vi "run s4gei state mach.vi"(8 "error in (no error)":errorcluster, 11 "S4GEI in":refnum<class "S4GEI.lvclass">) -> (0 "error out":errorcluster, 3 "S4GEI out":refnum<class "S4GEI.lvclass">)   [LabVIEW 2018, in "S4GEI.lvclass"]
uses:
  S4GEI.lvclass
  S4GEI.lvclass/S4GEI.ctl
  State Machine/State Machine.lvclass
  Channel GUI/Channel.lvclass
panel:
  out "preset modes":T1
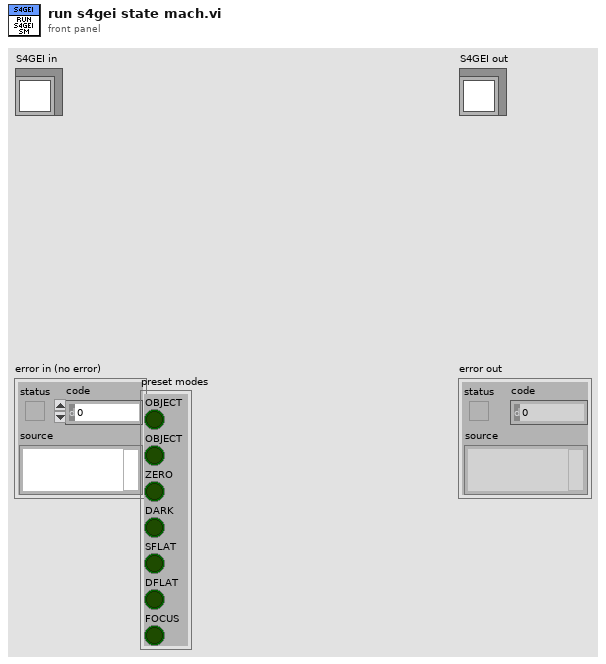
[diagram p1: front panel]
types:
  T1 = cluster{"OBJECT":bool, "OBJECT":bool, "ZERO":bool, "DARK":bool, "SFLAT":bool, "DFLAT":bool, "FOCUS":bool}
  T2 = cluster{"OBJECT":bool, "TEST":bool, "ZERO":bool, "DARK":bool, "SFLAT":bool, "DFLAT":bool, "FOCUS":bool}
  T3 = cluster{"OBJECT":string, "OBSERVER":string, "CTRLINTE":string, "PROJID":string, "SYNCMODE":string, "INSTMODE":string, "FILTER":string, "OBSTYPE":string, "GUIVRSN":string, "COMMENT":string, "broker":string, "timestamp":string, "CHANNEL 1":bool, "CHANNEL 2":bool, "CHANNEL 3":bool, "CHANNEL 4":bool, "TCSMODE":bool}
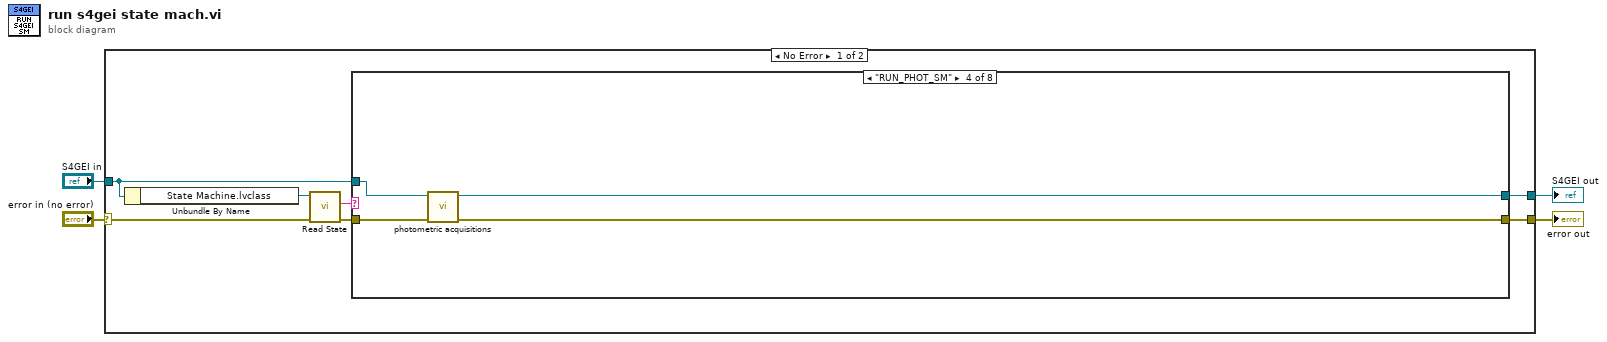
[diagram p0: block diagram]
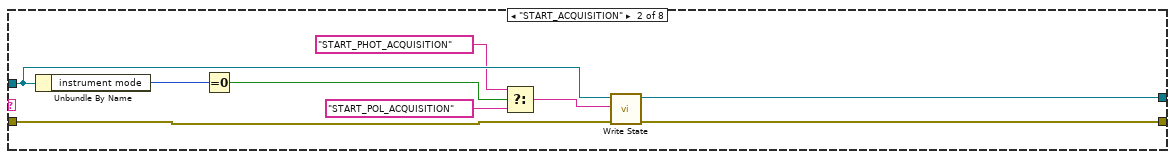
[diagram p3: hidden frame]
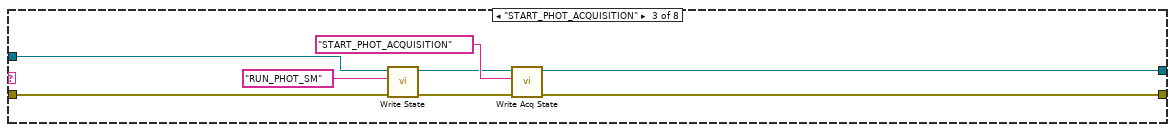
[diagram p4: hidden frame]
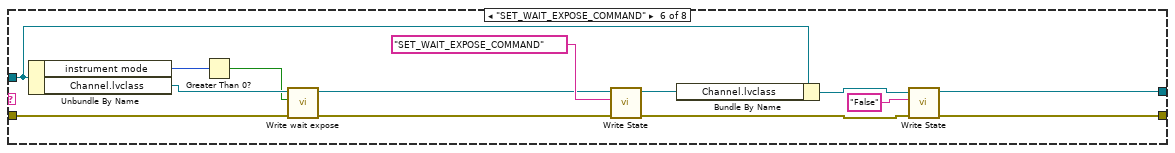
[diagram p6: hidden frame]
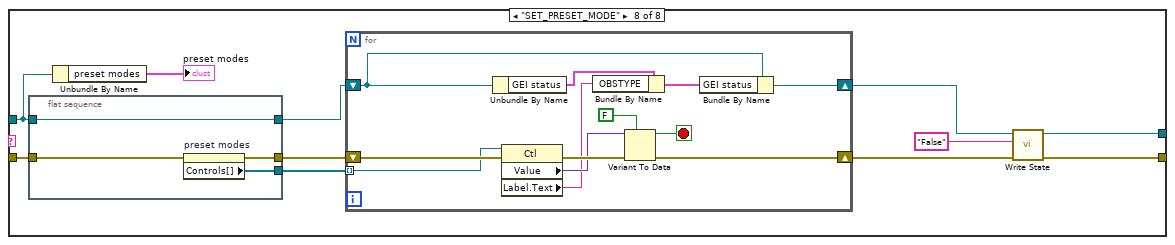
[diagram p8: hidden frame]
diagram:
  n1 = case shown="No Error" "error in (no error)" {
    selector: "error in (no error)" -> [w7 w81]
    tunnel: [w10 w81] -> w3
    tunnel: [w11 w80] -> w1
    tunnel: "S4GEI in" -> [w9 w80]
    frame No Error {
      n2 = Unbundle By Name(w9) -> ("State Machine.lvclass"=w8:refnum<class "State Machine.lvclass">)
      n3 = call-dynamic "Read State.vi"("error in (no error)"=w7, "State Machine in"=w8) -> ("error out"=w6:errorcluster, "State"=w5:string)  [unwired: 7 in, 1 out]
      n4 = case shown="\"RUN_PHOT_SM\"" w5 {
        tunnel: w9 -> [w13 w18 w27 w34 w36 w50 w52 w59]
        tunnel: w6 -> [w12 w19 w24 w31 w35 w39 w51 w58]
        tunnel: [w13 w21 w29 w33 w36 w47 w52 w56] -> w11
        tunnel: [w12 w22 w30 w32 w35 w46 w51 w57] -> w10
        frame "False", Default {
        }
        frame "START_ACQUISITION" {
          n5 = Unbundle By Name(w18) -> ("instrument mode"=w20:u16)
          n6 = Equal To 0?(x=w20) -> (x = 0?=w17:bool)
          n7 = Select(t="START_PHOT_ACQUISITION", s=w17, f="START_POL_ACQUISITION") -> (s? t:f=w15:string)
          n8 = call "Write State.vi"("error in (no error)"=w19, "State"=w15, "SPARC4_GEI in"=w18) -> ("error out"=w22:errorcluster, "SPARC4_GEI out"=w21:refnum<class "S4GEI.lvclass">)  [unwired: 7 in]
        }
        frame "START_PHOT_ACQUISITION" {
          n9 = call "Write State.vi"("error in (no error)"=w24, "State"="RUN_PHOT_SM", "SPARC4_GEI in"=w27) -> ("error out"=w25:errorcluster, "SPARC4_GEI out"=w26:refnum<class "S4GEI.lvclass">)  [unwired: 7 in]
          n10 = call "Write Acq State.vi"("error in (no error)"=w25, "State"="START_PHOT_ACQUISITION", "SPARC4_GEI in"=w26) -> ("error out"=w30:errorcluster, "SPARC4_GEI out"=w29:refnum<class "S4GEI.lvclass">)  [unwired: 7 in]
        }
        frame "RUN_PHOT_SM" {
          n11 = call "photometric acquisitions.vi"("error in (no error)"=w31, "S4GEI in"=w34) -> ("error out"=w32:errorcluster, "S4GEI out"=w33:refnum<class "S4GEI.lvclass">)  [unwired: 8 in]
        }
        frame "-------------------------" {
        }
        frame "SET_WAIT_EXPOSE_COMMAND" {
          n12 = Unbundle By Name(w50) -> ("instrument mode"=w38:u16, "Channel.lvclass"=w42:refnum<class "Channel.lvclass">)
          n13 = Greater Than 0?(x=w38) -> (x > 0?=w37:bool)
          n14 = call-dynamic "Write wait expose.vi"("error in (no error)"=w39, "wait expose"=w37, "Channel in"=w42) -> ("error out"=w40:errorcluster, "Channel out"=w41:refnum<class "Channel.lvclass">)  [unwired: 7 in]
          n15 = call "Write State.vi"("error in (no error)"=w40, "State"="SET_WAIT_EXPOSE_COMMAND", "Channel GEI in"=w41) -> ("error out"=w45:errorcluster, "Channel GEI out"=w49:refnum<class "Channel.lvclass">)  [unwired: 7 in]
          n16 = Bundle By Name(cluster=w50, "Channel.lvclass"=w49) -> (w48:refnum<class "S4GEI.lvclass">)
          n17 = call "Write State.vi"("error in (no error)"=w45, "State"="False", "SPARC4_GEI in"=w48) -> ("error out"=w46:errorcluster, "SPARC4_GEI out"=w47:refnum<class "S4GEI.lvclass">)  [unwired: 7 in]
        }
        frame "--------------------------" {
        }
        frame "SET_PRESET_MODE" {
          n18 = flat-sequence {
            tunnel: w58 -> [w65]
            tunnel: [w66] -> w63
            tunnel: w59 -> [w67]
            tunnel: [w67] -> w62
            tunnel: [w64] -> w60
            frame #0 {
              n19 = property on="preset modes" class="Clust (strict)"(error in=w65) -> (error out=w66:errorcluster, "Controls[]"=w64:refnum<vi>[])  [unwired: 1 in, 1 out]
            }
          }
          n20 = Unbundle By Name(w59) -> ("preset modes"=→"preset modes":T2)
          n21 = for {
            shift-right: [w70] -> w55
            shift-left: w62 -> [w74]
            shift-right: [w69] -> w54
            shift-left: w63 -> [w79]
            tunnel: w60 -> [w68] mode=indexing
            stop <- w75 stop-if-true
            n22 = Unbundle By Name(w74) -> ("GEI status"=w73:T3)
            n23 = property class="Ctl"(reference=w68, error in=w79) -> (error out=w78:errorcluster, "Value"=w77:variant, "Label.Text"=w71:string)  [unwired: 1 out]
            n24 = Bundle By Name(cluster=w73, "OBSTYPE"=w71) -> (w72:T3)
            n25 = Variant To Data(error in=w78, type=FALSE, Variant=w77) -> (data=w75:bool, error out=w69:errorcluster)
            n26 = Bundle By Name(cluster=w74, "GEI status"=w72) -> (w70:refnum<class "S4GEI.lvclass">)
          }
          n27 = call "Write State.vi"("error in (no error)"=w54, "State"="False" ("x"), "SPARC4_GEI in"=w55) -> ("error out"=w57:errorcluster, "SPARC4_GEI out"=w56:refnum<class "S4GEI.lvclass">)  [unwired: 7 in]
        }
      }
    }
    frame Error {
    }
  }
  "error out" <- w3
  "S4GEI out" <- w1
